vi "Create Default Configuration.vi"(0 "Sinks":refnum<class "Sink.lvclass">[](array[class]), 2 "Debug Level in":T1=enum."DEBUG", 3 "error in (no error)":errorcluster) -> (10 "error out":errorcluster)   [LabVIEW 2020, in "LV Log.lvlib"]
uses:
  LV Log.lvlib
  Sinks/Sink/Sink.lvclass
  Type Defs/Debug Level.ctl
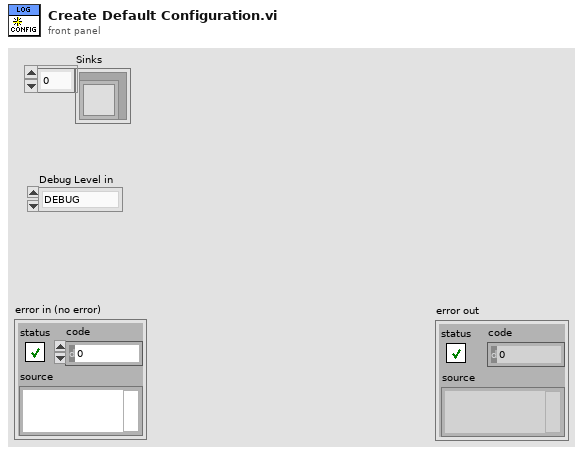
[diagram p1: front panel]
types:
  T1 = typedef "LV Log.lvlib/Debug Level.ctl" = enum16{"DEFAULT", "DEBUG", "INFO", "WARN", "ERROR", "FATAL"}
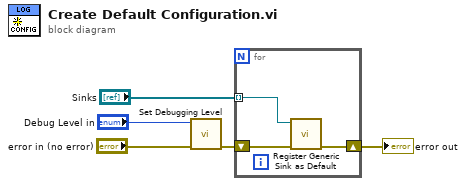
[diagram p0: block diagram]
diagram:
  n1 = call "Set Debugging Level.vi"("error in (no error)"="error in (no error)", "Debug Level in"="Debug Level in") -> ("error out"=w5:errorcluster)  [unwired: 9 in]
  n2 = for {
    tunnel: "Sinks" -> [w6] mode=indexing
    shift-right: [w7] -> w3
    shift-left: w5 -> [w8]
    n3 = call "Register Generic Sink as Default.vi"("error in (no error)"=w8, "Sink"=w6) -> ("error out"=w7:errorcluster)  [unwired: 9 in]
  }
  "error out" <- w3
